vi "Main_Console.vi"(0 "Value_In":string="0" caption="Value In", 5 "Command":T1(ring), 7 "Log_File_Folder":path=path "D:/Project Git file/Assignments/Assignment-4/Assignment-4.1/Assignment-4.1-LV21V/CSV" caption="Log File Folder", 9 "Stop":bool) -> (4 "Value_Out":string caption="Value Out")   [LabVIEW 2023]
doc: "This VI is the Console VI which communicate with Sour_Meas_instrument."
uses:
  <vilib>/Utility/file.llb/Write Delimited Spreadsheet (string).vi
panel:
  out "Error_Out":errorcluster
  in  "Error_In":errorcluster
  # "Control"
  # "Display"
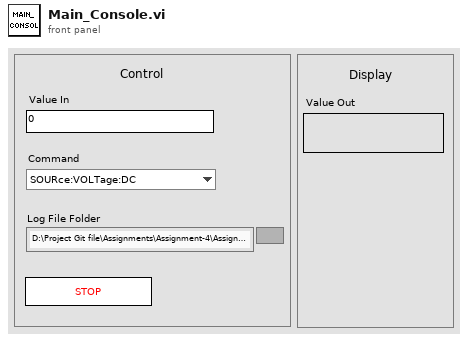
[diagram p1: front panel]
types:
  T1 = enum16{"SOURce:VOLTage:DC", "SOURce:CURRent:DC", "MEASure:VOLTage:DC?", "MEASure:CURRent:DC?"}
  T2 = enum16{"Left Button", "Center Button", "Right Button", "Window Close"}
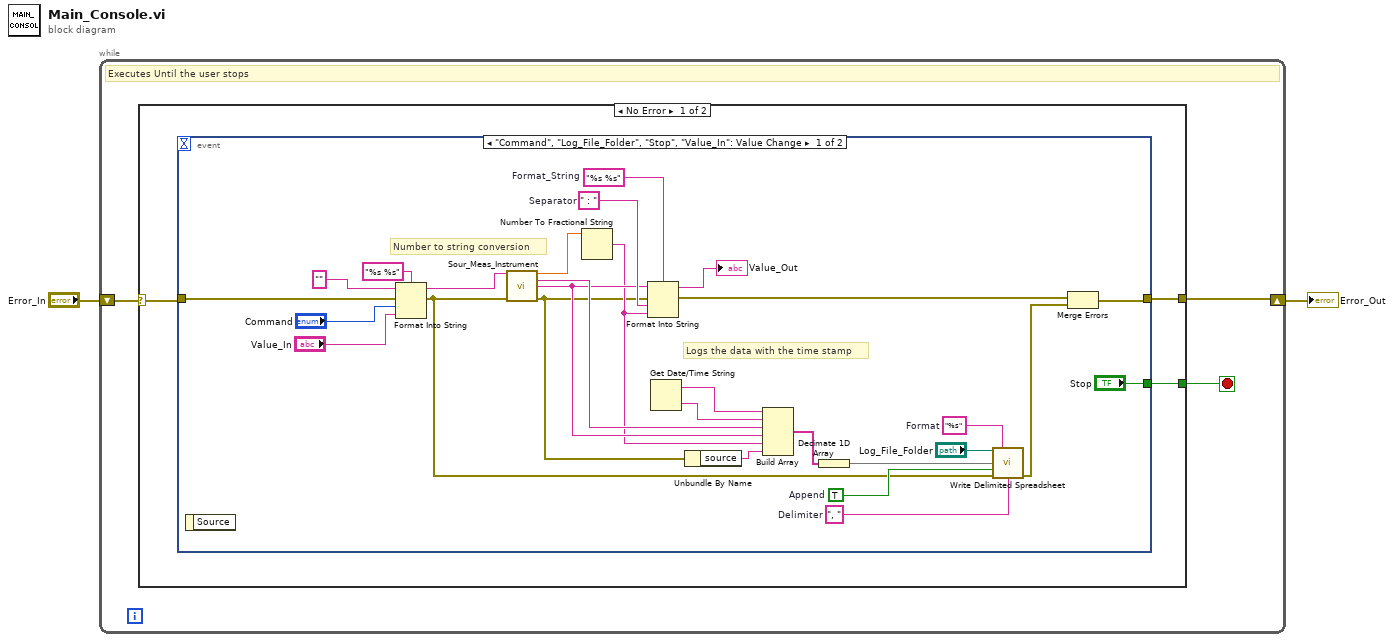
[diagram p0: block diagram]
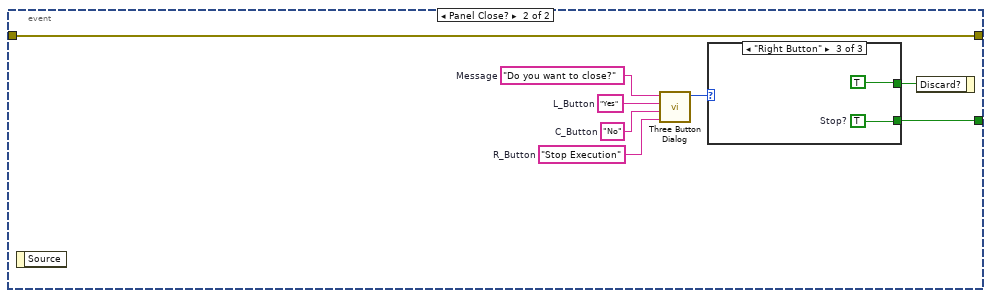
[diagram p2: hidden frame]
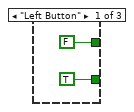
[diagram p3: hidden frame]
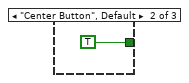
[diagram p4: hidden frame]
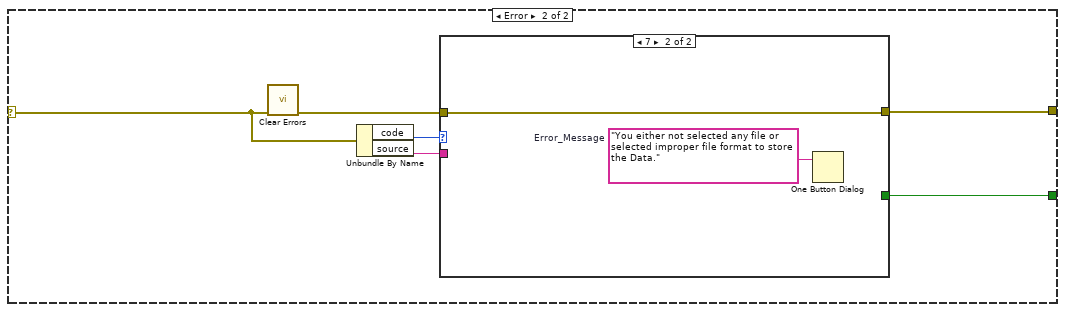
[diagram p5: hidden frame]
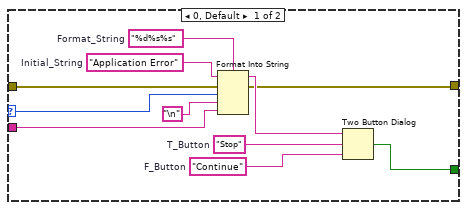
[diagram p6: hidden frame]
diagram:
  n1 = while {
    shift-right: [w3] -> w1
    shift-left: "Error_In" -> [w4]
    stop <- w5 stop-if-true
    # "Executes Until the user stops"
    n2 = case shown="No Error" w4 {
      selector: w4 -> [w7 w55]
      tunnel: [w8 w52] -> w5
      tunnel: [w6 w50] -> w3
      frame No Error {
        n3 = event shown="[0] \"Command\", \"Log_File_Folder\", \"Stop\", \"Value_In\": Value Change" {
          selector: _ -> [_ _]
          dyn-events: _ -> [_ _]
          timeout: _ -> [_ _]
          tunnel: ["Stop" w38] -> w8
          tunnel: w7 -> [w12 w37]
          tunnel: [w11 w37] -> w6
          event "Command", "Log_File_Folder", "Stop", "Value_In": Value Change {
            w27 = TRUE  # Append
            w33 = "%s"  # Format
            w24 = ", "  # Delimiter
            w34 = " : "  # Separator
            w35 = "%s %s"  # Format_String
            # "Number to string conversion"
            # "Logs the data with the time stamp"
            n4 = event-data() -> ()  [unwired: 1 in, 1 out]
            n5 = Format Into String(format string="%s %s", initial string="", error in=w12, "Command", "Value_In") -> (resulting string=w14:string, error out=w13:errorcluster)
            n6 = call "Sour_Meas_Instrument.vi"("Command"=w14, "Error_In"=w13) -> ("Responce"=w36:dbl, "Action"=w32:string, "Parameter"=w31:string, "Error_Out"=w19:errorcluster)  [unwired: 10 in]
            n7 = Number To Fractional String(number=w36) -> (F-format string=w30:string)  [unwired: 3 in]
            n8 = Format Into String(format string=w35, initial string=w31, error in=w19, w34, w30) -> (resulting string=→"Value_Out":string, error out=w22:errorcluster)
            n9 = Get Date/Time String() -> (date string=w26:string, time string=w25:string)  [unwired: 3 in]
            n10 = Unbundle By Name(w19) -> ("source"=w20:string)
            n11 = Build Array(w26, w25, w32, w31, w30, w20) -> (w29:string[])
            n12 = Decimate 1D Array(w29) -> (w28:string[])
            n13 = call-poly <vilib>:"Write Delimited Spreadsheet.vi"("file path (dialog if empty)"="Log_File_Folder", "format (%s)"=w33, "1D data"=w28, "append to file? (new file:F)"=w27, "error in (no error)"=w13, "delimiter (\\t)"=w24) -> ("error out"=w23:errorcluster)  [unwired: 8 in, 1 out]
            n14 = Merge Errors(w22, w23) -> (w11:errorcluster)
          }
          event Panel Close? {
            w41 = "Stop Execution"  # R_Button
            w42 = "No"  # C_Button
            w43 = "Yes"  # L_Button
            w44 = "Do you want to close?"  # Message
            n15 = event-data() -> ()  [unwired: 1 in, 1 out]
            n16 = call <vilib>:"Three Button Dialog.vi"("Right Button Text (\"Cancel\")"=w41, "Center Button Text (\"No\")"=w42, "Left Button Text (\"Yes\")"=w43, "message"=w44) -> ("Which Button?"=w40:T2)  [unwired: 7 in]
            n17 = case shown="\"Right Button\"" w40 {
              tunnel: [FALSE TRUE TRUE] -> w39
              tunnel: [TRUE _ w49] -> w38
              frame "Left Button" {
              }
              frame "Center Button", Default {
              }
              frame "Right Button" {
                w49 = TRUE  # Stop?
              }
            }
            n18 = event-data ("Event Filter Node")("Discard?"=w39) -> ()  [unwired: 1 in, 1 out]
          }
        }
      }
      frame Error {
        n19 = call <vilib>:"Clear Errors.vi"("error in (no error)"=w55) -> ("error out"=w51:errorcluster)  [unwired: 5 in, 1 out]
        n20 = Unbundle By Name(w55) -> ("code"=w54:i32, "source"=w53:string)
        n21 = case shown="7" w54 {
          selector: w54 -> [w66 _]
          tunnel: w53 -> [w61 _]
          tunnel: [w62 _] -> w52
          tunnel: w51 -> [w59 w67]
          tunnel: [w58 w67] -> w50
          frame 0, Default {
            w57 = "%d%s%s"  # Format_String
            w60 = "Application Error"  # Initial_String
            w63 = "Stop"  # T_Button
            w64 = "Continue"  # F_Button
            n22 = Format Into String(format string=w57, initial string=w60, error in=w59, w66, "\n", w61) -> (resulting string=w65:string, error out=w58:errorcluster)
            n23 = Two Button Dialog(message=w65, 1:w64, 2:w63) -> (T button?=w62:bool)
          }
          frame 7 {
            w68 = "You either not selected any file or selected improper file format to store the Data."  # Error_Message
            n24 = One Button Dialog(message=w68) -> ()  [unwired: 1 in, 1 out]
          }
        }
      }
    }
  }
  "Error_Out" <- w1
